vi "Search Item by ID.vi"(9 "Item ID":string, 11 "Items":refnum<class "Item.lvclass">[](array[class])) -> (1 "Index":i32, 3 "Item":refnum<class "Item.lvclass">)   [LabVIEW 2020, in "VI Properties Editor.lvlib"]
doc: "Searches <B>Items</B> for the item identified by <B>Item ID</B>."
uses:
  VI Properties Editor.lvlib
  Classes/Item/Item.lvclass
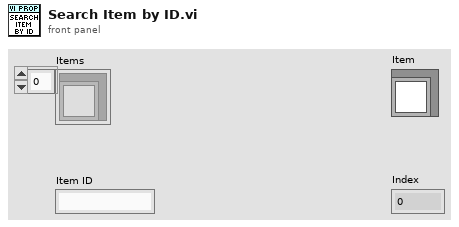
[diagram p1: front panel]
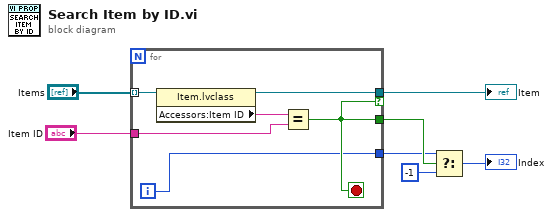
[diagram p0: block diagram]
diagram:
  n1 = for {
    tunnel: "Items" -> [w13] mode=indexing
    tunnel: "Item ID" -> [w11]
    tunnel: [w9] -> w5
    tunnel: [w10] -> w2 if=w9
    tunnel: [w8] -> w4
    i -> [w8]
    stop <- w9 stop-if-true
    n2 = property class="Item.lvclass"(reference=w13) -> (reference out=w10:refnum<class "Item.lvclass">, "Accessors:Item ID"=w12:string)  [unwired: 1 in, 1 out]
    n3 = Equal?(x=w12, y=w11) -> (x = y?=w9:bool)
  }
  "Item" <- w2
  n4 = Select(t=w4, s=w5, f=-1) -> (s? t:f=→"Index":i32)
